vi "SetMultipleTiles.vi"(8 "error in (no error)":errorcluster, 9 "TileCodes":string[][](array[string]), 10 "Position":T1, 11 "Game in":refnum<class "Game.lvclass">) -> (0 "error out":errorcluster, 3 "Game out":refnum<class "Game.lvclass">)   [LabVIEW 2019, in "RT_Game.lvlib" / "Game.lvclass"]
uses:
  Game.lvclass
  Coordinate.ctl
  Game.lvclass/Game.ctl
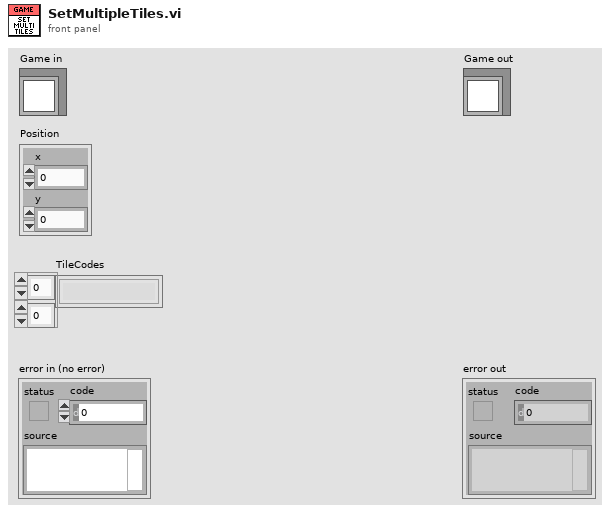
[diagram p1: front panel]
types:
  T1 = typedef "RT_Game.lvlib/Game.lvclass/Coordinate.ctl" = cluster{"x":dbl, "y":dbl}
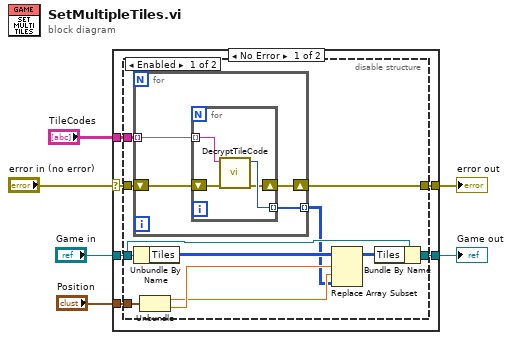
[diagram p0: block diagram]
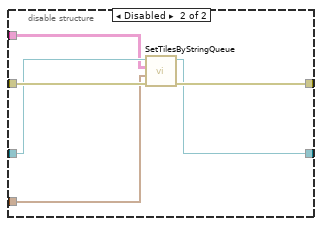
[diagram p2: hidden frame]
diagram:
  n1 = case shown="No Error" "error in (no error)" {
    selector: "error in (no error)" -> [w7 w39]
    tunnel: [w8 w39] -> w5
    tunnel: [w11 w38] -> w3
    tunnel: "Game in" -> [w12 w38]
    tunnel: "Position" -> [w10 _]
    tunnel: "TileCodes" -> [w9 _]
    frame No Error {
      n2 = disable-structure shown="Enabled" {
        disable-tunnel: w12 -> [w23 w35]
        disable-tunnel: [w22 w34] -> w11
        disable-tunnel: w10 -> [w21 w32]
        disable-tunnel: w9 -> [w20 w33]
        disable-tunnel: [w19 w36] -> w8
        disable-tunnel: w7 -> [w18 w37]
        frame Enabled {
          n3 = for {
            tunnel: w20 -> [w27] mode=indexing
            tunnel: [w26] -> w13 mode=indexing
            shift-right: [w25] -> w19
            shift-left: w18 -> [w24]
            n4 = for {
              tunnel: w27 -> [w31] mode=indexing
              tunnel: [w30] -> w26 mode=indexing
              shift-right: [w29] -> w25
              shift-left: w24 -> [w28]
              n5 = call "DecryptTileCode.vi"("error in (no error)"=w28, "TileCode"=w31) -> ("error out"=w29:errorcluster, "TileCode"=w30:u16)  [unwired: 6 in, 2 out]
            }
          }
          n6 = Unbundle By Name(w23) -> ("Tiles"=w15:u16[][])
          n7 = Unbundle(w21) -> ("x"=w16:dbl, "y"=w17:dbl)
          n8 = Replace Array Subset(array=w15, new element=w13, index (row)=w17, index (col)=w16) -> (w14:u16[][])
          n9 = Bundle By Name(cluster=w23, "Tiles"=w14) -> (w22:refnum<class "Game.lvclass">)
        }
        frame Disabled {
          n10 = call "SetTilesByStringQueue.vi"("error in (no error)"=w37, "Position"=w32, "TileStrings"=w33, "Game in"=w35) -> ("error out"=w36:errorcluster, "Game out"=w34:refnum<class "Game.lvclass">)  [unwired: 6 in]
        }
      }
    }
    frame Error {
    }
  }
  "error out" <- w5
  "Game out" <- w3
